vi "Fetch (Multiple).vi"(4 "Buffer Element2 ()":i32(ring) items=["", "Date", "Extra", "Formatted", "Fractional", "Reading", "Relative", "Seconds", "Status", "Time", "Tstamp", "Unit", "CHAN", "Extra Form", "Extra Unit"], 5 "Sample Count (0)":i32, 6 "Buffer Element1 ()":i32(ring) items=["", "Date", "Extra", "Formatted", "Fractional", "Reading", "Relative", "Seconds", "Status", "Time", "Tstamp", "Unit", "CHAN", "Extra Format", "Extra Unit"], 7 "Timeout (100000 ms)":i32=100000, 8 "error in (no error)":errorcluster, 9 "Buffer Name ()":string, 11 "VISA resource name":refnum<visa-resource-name>) -> (0 "error out":errorcluster, 2 "Measurements":dbl[](array[numeric]), 3 "VISA resource name out":refnum<visa-resource-name>)   [LabVIEW 2016, in "Keithley DMM6500 DAQ6500 Series.lvlib"]
doc: "Reads and returns multiple measurements from the instrument. Use this VI when you want to take multiple measurements using an immediate trigger. Use the low-level VIs for other triggering options."
uses:
  Keithley DMM6500 DAQ6500 Series.lvlib
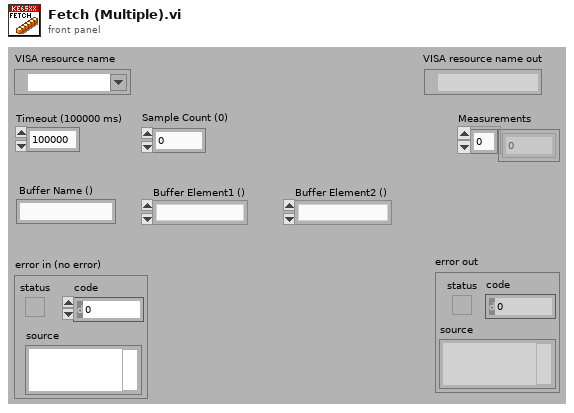
[diagram p1: front panel]
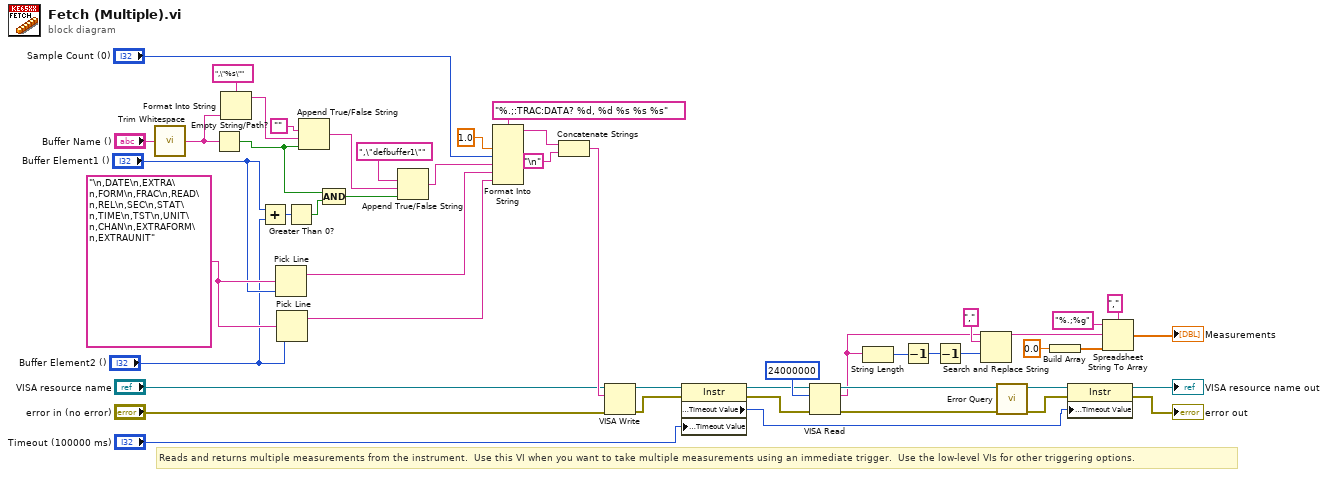
[diagram p0: block diagram]
diagram:
  w11 = "\n,DATE\n,EXTRA\n,FORM\n,FRAC\n,READ\n,REL\n,SEC\n,STAT\n,TIME\n,TST\n,UNIT\n,CHAN\n,EXTRAFORM\n,EXTRAUNIT" ("multi-line string")
  # "Reads and returns multiple measurements from the instrument.  Use this VI when you want to take multiple measurements using an immediate trigger.  Use the low-level VIs for other triggering options."
  n1 = call <vilib>:"Trim Whitespace.vi"("string"="Buffer Name ()") -> ("trimmed string"=w2:string)  [unwired: 1 in]
  n2 = Empty String/Path?(string/path=w2) -> (empty?=w1:bool)
  n3 = Format Into String(format string=",\"%s\"", w2) -> (resulting string=w42:string)  [unwired: 2 in, 1 out]
  n4 = Add(x="Buffer Element1 ()", y="Buffer Element2 ()") -> (x+y=w4:i32)
  n5 = Pick Line(multi-line string=w11, line index="Buffer Element1 ()") -> (output string=w13:string)  [unwired: 1 in]
  n6 = Pick Line(multi-line string=w11, line index="Buffer Element2 ()") -> (output string=w12:string)  [unwired: 1 in]
  n7 = Greater Than 0?(x=w4) -> (x > 0?=w3:bool)
  n8 = Append True/False String(1:w1, 2:w42, 3:"") -> (0:w6:string)  [unwired: 1 in]
  n9 = Compound Arithmetic op=AND(w1, w3) -> (w7:bool)
  n10 = Append True/False String(1:w7, 2:w6, 3:",\"defbuffer1\"" ("true string")) -> (0:w8:string)  [unwired: 1 in]
  n11 = Format Into String(format string="%.;:TRAC:DATA? %d, %d %s %s %s", 1.0 ("input 1"), "Sample Count (0)", w8, w13, w12) -> (resulting string=w19:string)  [unwired: 2 in, 1 out]
  n12 = Concatenate Strings(w19, "\n") -> (w46:string)
  n13 = VISA Write(VISA resource name="VISA resource name", write buffer=w46, error in (no error)="error in (no error)") -> (VISA resource name out=w29:refnum<visa-resource-name>, error out=w28:errorcluster)  [unwired: 1 out]
  n14 = property on="Property Node" class="Instr"(reference=w29, error in=w28, "General Settings:Timeout Value"="Timeout (100000 ms)") -> (reference out=w26:refnum<visa-resource-name>, error out=w27:errorcluster, "General Settings:Timeout Value"=w21:u32)
  n15 = VISA Read(VISA resource name=w26, byte count=i64 24000000, error in (no error)=w27) -> (VISA resource name out=w48:refnum<visa-resource-name>, read buffer=w31:string, error out=w47:errorcluster)  [unwired: 1 out]
  n16 = String Length(string=w31) -> (length=w34:i32)
  n17 = Decrement(x=w34) -> (x-1=w32:i32)
  n18 = Decrement(x=w32) -> (x-1=w33:i32)
  n19 = Search and Replace String(input string=w31, search string=",", offset=w33) -> (result string=w37:string)  [unwired: 5 in, 3 out]
  n20 = call "Error Query.vi"("error in (no error)"=w47, "VISA resource name"=w48) -> ("error out"=w23:errorcluster, "VISA resource name out"=w25:refnum<visa-resource-name>)  [unwired: 6 in, 2 out]
  n21 = Build Array(0.0 ("element")) -> (w40:dbl[])
  n22 = property on="Property Node" class="Instr"(reference=w25, error in=w23, "General Settings:Timeout Value"=w21) -> (reference out=→"VISA resource name out":refnum<visa-resource-name>, error out=→"error out":errorcluster)
  n23 = Spreadsheet String To Array(delimiter (Tab)=",", format string="%.;%g", spreadsheet string=w37, array type (2D Dbl)=w40) -> (array=→"Measurements":dbl[])
